vi "GT_server_v2.vi"() -> ()   [LabVIEW 2010]
uses:
  <vilib>/Motion/FlexMotion/CustomControls/CustomControls.llb/Axis To Control.flx
  <vilib>/Motion/FlexMotion/CustomControls/CustomControls.llb/Axis # (8 axes).flx
  <vilib>/Motion/FlexMotion/FunctionsVIs/MotionIO.llb/Enable Home Inputs (8 axes).flx
  <vilib>/Motion/FlexMotion/FunctionsVIs/StartStopMotion.llb/Start Motion (8 axes).flx
panel:
  out "Position 3":i32
  in  "stop":bool
  in  "Board ID":T1=1 min=1 max=32 step=1
  out "Position 2":i32
  in  "port":u16=2525
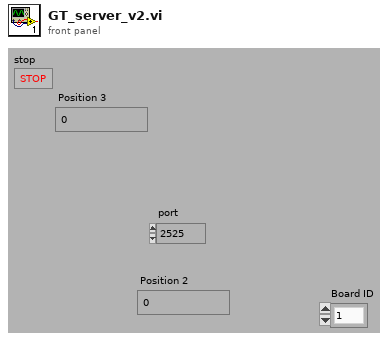
[diagram p1: front panel]
types:
  T1 = typedef "Board Id" = u8
  T2 = typedef "Axis To Control.flx" = u16
  T3 = typedef "Bd Id Out" = u8
  T4 = typedef "Resource Out (Enum).flx" = u16
  T5 = enum16{"Standard", "Buffered", "CRLF", "Immediate"}
  T6 = typedef "Axis # (8 axes).flx" = cluster{"1":bool, "2":bool, "3":bool, "4":bool, "5":bool, "6":bool, "7":bool, "8":bool}
  T7 = enum16{"Home", "Index", "Center", "Forward Limit", "Reverse Limit", "Run Sequence"}
  T8 = enum16{"Absolute Position", "Relative Position", "Velocity", "Relative to Cap Pos", "Modulus Position", "Absolute Contouring", "Relative Contouring"}
  T9 = typedef "AxisOrVectorSpaceControl To Control.flx" = u16
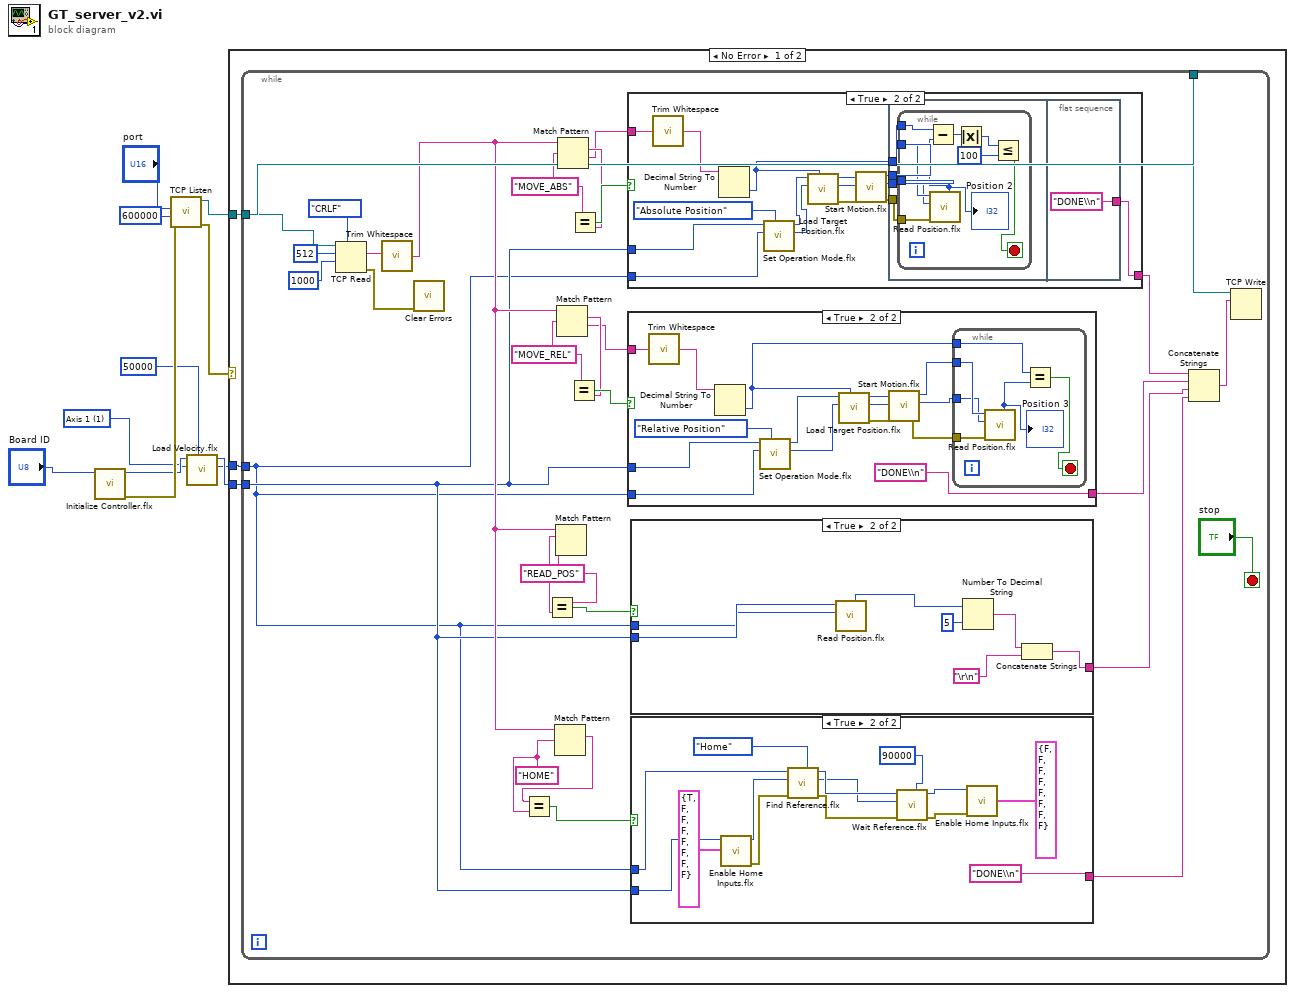
[diagram p0: block diagram]
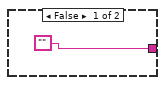
[diagram p2: hidden frame]
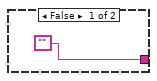
[diagram p3: hidden frame]
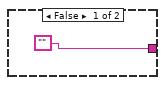
[diagram p4: hidden frame]
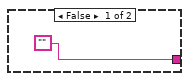
[diagram p5: hidden frame]
diagram:
  w3 = T2 1 items=["Axis 1"=1, "Axis 2"=2, "Axis 3"=3, "Axis 4"=4, "Axis 5"=5, "Axis 6"=6, "Axis 7"=7, "Axis 8"=8] ("Axis")
  n1 = call <vilib>:"Initialize Controller.flx"("Board ID"="Board ID") -> ("error out"=w7:errorcluster, "Bd ID Out"=w5:T3)  [unwired: 7 in]
  n2 = call <vilib>:"TCP Listen.vi"("error in (no error)"=w7, "timeout ms (wait forever: -1)"=600000, "port"="port") -> ("error out"=w9:errorcluster, "connection ID"=w8:refnum<k5>)  [unwired: 5 in, 2 out]
  n3 = call <vilib>:"Load Velocity.flx"("Velocity (10000)"=50000, "Axis or Vector Space"=w3, "Board ID"=w5) -> ("Resource Output"=w2:T4, "Bd ID Out"=w4:T3)  [unwired: 4 in, 1 out]
  n4 = case shown="No Error" w9 {
    tunnel: w8 -> [w12 _]
    tunnel: w4 -> [w14 _]
    tunnel: w2 -> [w13 _]
    frame No Error {
      n5 = while {
        tunnel: w12 -> [w30]
        tunnel: w14 -> [w16]
        tunnel: w13 -> [w15]
        tunnel: w12 -> [w31]
        stop <- "stop" stop-if-true
        w19 = "HOME" ("regular expression")
        w25 = "MOVE_REL" ("regular expression")
        w40 = "READ_POS" ("regular expression")
        w37 = "MOVE_ABS" ("regular expression")
        n6 = TCP Read(connection ID=w31, bytes to read=512, 7:T5."CRLF" ("mode (standard)"), 9:1000 ("timeout ms (25000)")) -> (data out=w32:string, error out=w28:errorcluster)  [unwired: 1 in, 1 out]
        n7 = call <vilib>:"Trim Whitespace.vi"("string"=w32) -> ("trimmed string"=w21:string)  [unwired: 1 in]
        n8 = call <vilib>:"Clear Errors.vi"("error in (no error)"=w28) -> ()  [unwired: 6 in, 1 out]
        n9 = Match Pattern(string=w21, regular expression=w19) -> (match substring=w20:string)  [unwired: 1 in, 3 out]
        n10 = Equal?(x=w20, y=w19) -> (x = y?=w18:bool)
        n11 = Match Pattern(string=w21, regular expression=w40) -> (match substring=w41:string)  [unwired: 1 in, 3 out]
        n12 = Equal?(x=w40, y=w41) -> (x = y?=w42:bool)
        n13 = Match Pattern(string=w21, regular expression=w25) -> (match substring=w26:string, after substring=w24:string)  [unwired: 1 in, 2 out]
        n14 = Match Pattern(string=w21, regular expression=w37) -> (match substring=w38:string, after substring=w36:string)  [unwired: 1 in, 2 out]
        n15 = Equal?(x=w25, y=w26) -> (x = y?=w27:bool)
        n16 = Equal?(x=w37, y=w38) -> (x = y?=w39:bool)
        n17 = case shown="True" w39 {
          tunnel: w36 -> [_ w105]
          tunnel: ["" w91] -> w43
          tunnel: w16 -> [_ w94]
          tunnel: w15 -> [_ w93]
          frame False {
          }
          frame True {
            n18 = call <vilib>:"Trim Whitespace.vi"("string"=w105) -> ("trimmed string"=w104:string)  [unwired: 1 in]
            n19 = Decimal String To Number(string=w104) -> (number=w97:i32)  [unwired: 2 in, 1 out]
            n20 = call <vilib>:"Set Operation Mode.flx"("Position Mode (Absolute)"=T8."Absolute Position", "Axis or Vector Space"=w93, "Board ID"=w94) -> ("Resource Output"=w95:T4, "Bd ID Out"=w96:T3)  [unwired: 3 in, 1 out]
            n21 = call <vilib>:"Load Target Position.flx"("Target Position (0)"=w97, "Axis"=w95, "Board ID"=w96) -> ("error out"=w103:errorcluster, "Resource Output"=w101:T4, "Bd ID Out"=w102:T3)  [unwired: 4 in]
            n22 = call-poly <vilib>:"Start Motion.flx"("error in (no error)"=w103, "Axis or Vector Space"=w101, "Board ID"=w102) -> ("error out"=w98:errorcluster, "Resource Output"=w99:T4, "Bd ID Out"=w100:T3)  [unwired: 3 in]
            n23 = flat-sequence {
              tunnel: w100 -> [w109]
              tunnel: w99 -> [w108]
              tunnel: w98 -> [w107]
              tunnel: w97 -> [w106]
              tunnel: ["DONE\\n"] -> w91
              frame #0 {
                n24 = while {
                  tunnel: w109 -> [w118]
                  tunnel: w108 -> [w117]
                  tunnel: w107 -> [w116]
                  tunnel: w106 -> [w113]
                  stop <- w114 stop-if-true
                  n25 = call <vilib>:"Read Position.flx"("error in (no error)"=w116, "Axis"=w117, "Board ID"=w118) -> ("Position"=w115:i32)  [unwired: 3 in, 3 out]
                  "Position 2" <- w115
                  n26 = Subtract(x=w113, y=w115) -> (x-y=w112:i32)
                  n27 = Absolute Value(x=w112) -> (abs(x)=w111:i32)
                  n28 = Less Or Equal?(x=w111, y=100) -> (x <= y?=w114:bool)
                }
              }
              frame #1 {
              }
            }
          }
        }
        n29 = case shown="True" w27 {
          tunnel: w24 -> [_ w75]
          tunnel: ["" "DONE\\n"] -> w22
          tunnel: w16 -> [_ w63]
          tunnel: w15 -> [_ w62]
          frame False {
          }
          frame True {
            n30 = call <vilib>:"Trim Whitespace.vi"("string"=w75) -> ("trimmed string"=w74:string)  [unwired: 1 in]
            n31 = Decimal String To Number(string=w74) -> (number=w67:i32)  [unwired: 2 in, 1 out]
            n32 = call <vilib>:"Set Operation Mode.flx"("Position Mode (Absolute)"=T8."Relative Position", "Axis or Vector Space"=w62, "Board ID"=w63) -> ("Resource Output"=w64:T4, "Bd ID Out"=w65:T3)  [unwired: 3 in, 1 out]
            n33 = call <vilib>:"Load Target Position.flx"("Target Position (0)"=w67, "Axis"=w64, "Board ID"=w65) -> ("error out"=w73:errorcluster, "Resource Output"=w71:T4, "Bd ID Out"=w72:T3)  [unwired: 4 in]
            n34 = call-poly <vilib>:"Start Motion.flx"("error in (no error)"=w73, "Axis or Vector Space"=w71, "Board ID"=w72) -> ("error out"=w68:errorcluster, "Resource Output"=w69:T4, "Bd ID Out"=w70:T3)  [unwired: 3 in]
            n35 = while {
              tunnel: w70 -> [w81]
              tunnel: w69 -> [w80]
              tunnel: w68 -> [w79]
              tunnel: w67 -> [w77]
              stop <- w76 stop-if-true
              n36 = call <vilib>:"Read Position.flx"("error in (no error)"=w79, "Axis"=w80, "Board ID"=w81) -> ("Position"=w78:i32)  [unwired: 3 in, 3 out]
              "Position 3" <- w78
              n37 = Equal?(x=w77, y=w78) -> (x = y?=w76:bool)
            }
          }
        }
        n38 = case shown="True" w42 {
          tunnel: ["" w86] -> w23
          tunnel: w16 -> [_ w85]
          tunnel: w15 -> [_ w84]
          frame False {
          }
          frame True {
            n39 = call <vilib>:"Read Position.flx"("Axis"=w84, "Board ID"=w85) -> ("Position"=w89:i32)  [unwired: 4 in, 3 out]
            n40 = Number To Decimal String(number=w89, width (-)=i16 5) -> (decimal integer string=w88:string)
            n41 = Concatenate Strings(w88, "\r\n") -> (w86:string)
          }
        }
        n42 = case shown="True" w18 {
          tunnel: ["" "DONE\\n"] -> w17
          tunnel: w16 -> [_ w50]
          tunnel: w15 -> [_ w57]
          frame False {
          }
          frame True {
            n43 = call-poly <vilib>:"Enable Home Inputs.flx"("Homes (Disabled)"=T6 {"1"=TRUE, "2"=FALSE, "3"=FALSE, "4"=FALSE, "5"=FALSE, "6"=FALSE, "7"=FALSE, "8"=FALSE}, "Board ID"=w50) -> ("error out"=w52:errorcluster, "Bd ID Out"=w51:T3)  [unwired: 5 in]
            n44 = call <vilib>:"Find Reference.flx"("Search Type"=T7."Home", "error in (no error)"=w52, "Axis or Vector Space"=w51, "Board ID"=w57) -> ("error out"=w53:errorcluster, "Axis or Vector Space Output"=w55:T9, "Bd ID Out"=w56:T3)  [unwired: 5 in]
            n45 = call <vilib>:"Wait Reference.flx"("Timeout (ms)"=u32 90000, "error in (no error)"=w53, "Axis or Vector Space"=w55, "Board ID"=w56) -> ("error out"=w48:errorcluster, "Bd ID Out"=w47:T3)  [unwired: 4 in, 2 out]
            n46 = call-poly <vilib>:"Enable Home Inputs.flx"("Homes (Disabled)"=T6 {"1"=FALSE, "2"=FALSE, "3"=FALSE, "4"=FALSE, "5"=FALSE, "6"=FALSE, "7"=FALSE, "8"=FALSE}, "error in (no error)"=w48, "Board ID"=w47) -> ()  [unwired: 4 in, 2 out]
          }
        }
        n47 = Concatenate Strings(w43, w22, w23, w17) -> (w44:string)
        n48 = TCP Write(connection ID=w30, data in=w44) -> ()  [unwired: 2 in, 3 out]
      }
    }
    frame Error {
    }
  }
